vi "Engine Out - GDI - EGR Actuation.vi"(11 "EGR Position Setpoint [%Open]":sgl) -> (3 "EGR LS Output":T1)   [LabVIEW 2015, in "ECS-RT.lvlib"]
uses:
  ECS-RT.lvlib
  Typedefs/Raw Outputs/LS.ctl
  ECS-Shared.lvlib
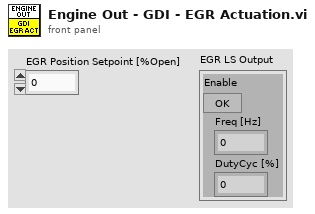
[diagram p1: front panel]
types:
  T1 = typedef "ECS-Shared.lvlib/LS.ctl" = cluster{"Enable":bool, "Freq [Hz]":sgl, "DutyCyc [%]":sgl}
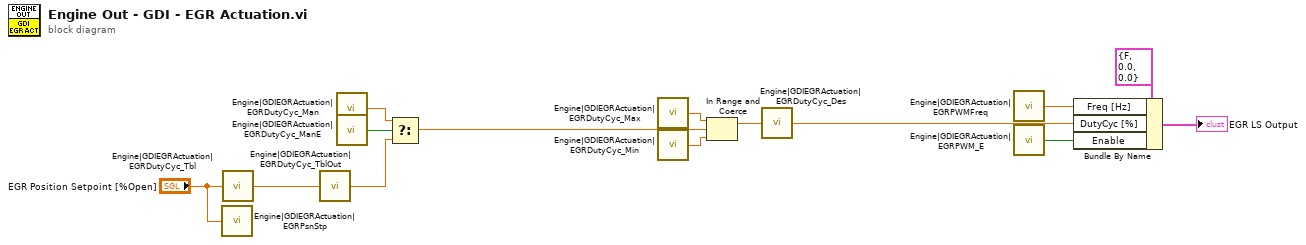
[diagram p0: block diagram]
diagram:
  n1 = call "Engine|GDIEGRActuation|EGRPsnStp"("Value"="EGR Position Setpoint [%Open]") -> ()
  n2 = call "Engine|GDIEGRActuation|EGRDutyCyc_Tbl"("X Index"="EGR Position Setpoint [%Open]") -> ("Y"=w3:sgl)
  n3 = call "Engine|GDIEGRActuation|EGRDutyCyc_TblOut"("Value"=w3) -> ()
  n4 = call "Engine|GDIEGRActuation|EGRDutyCyc_Man"() -> ("Value"=w6:sgl)
  n5 = call "Engine|GDIEGRActuation|EGRDutyCyc_ManE"() -> ("Value"=w7:bool)
  n6 = Select(t=w6, s=w7, f=w3) -> (s? t:f=w8:sgl)
  n7 = call "Engine|GDIEGRActuation|EGRDutyCyc_Max"() -> ("Value"=w9:sgl)
  n8 = call "Engine|GDIEGRActuation|EGRDutyCyc_Min"() -> ("Value"=w10:sgl)
  n9 = In Range and Coerce(upper limit=w9, x=w8, lower limit=w10) -> (coerced(x)=w2:sgl)  [unwired: 1 out]
  n10 = call "Engine|GDIEGRActuation|EGRDutyCyc_Des"("Value"=w2) -> ()
  n11 = call "Engine|GDIEGRActuation|EGRPWMFreq"() -> ("Value"=w12:sgl)
  n12 = call "Engine|GDIEGRActuation|EGRPWM_E"() -> ("Value"=w11:bool)
  n13 = Bundle By Name(cluster=T1 {"Enable"=FALSE, "Freq [Hz]"=0.0, "DutyCyc [%]"=0.0} ("LS Output"), "Freq [Hz]"=w12, "DutyCyc [%]"=w2, "Enable"=w11) -> (→"EGR LS Output":T1)
